vi "WSVCAP SHL Host LL Build SRL Set Voltage CMD.vi"(5 "Data out (14-bit)":u16 format="%04x", 6 "FPGA (Required for Vref = -1)":T1, 7 "Vref (-1: Unchanged)":dbl=-1.0 format="%.3f V", 8 "error in (no error)":errorcluster, 9 "Voltage (-1: Use Data Out)":dbl=-1.0 format="%.3f V", 10 "Channel (0-5)":u32, 11 "DUT":T2) -> (0 "error out":errorcluster, 1 "Raw CMD [Hex]":u32 max=5 step=1 format="0x%05x", 2 "Dev Idx (0-5)":u32, 3 "Raw CMD [Str]":string, 4 "Device Ch Idx (0-31)":u32)   [LabVIEW 2017]
uses:
  Type Defs/WSVCAP SHL DUT Number Enum.ctl
  Type Defs/WSVCAP SHL FPGA Enum.ctl
  Host SRL/Host SRL.lvlib
panel:
  out "Vref Used (V)":dbl format="%.3f V"
  out "D [U16]":u32 format="%.0x"
  out "Raw CMD [Bin]":u32 max=5 step=1 format="0b%019b"
  # "D = [Vout * (2^14)] / (50 * Vref)"
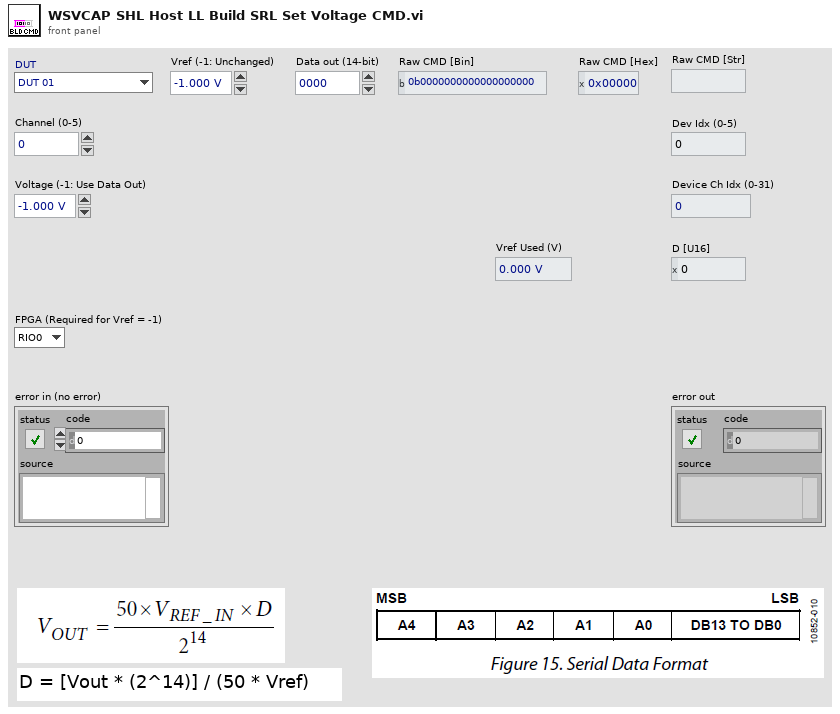
[diagram p1: front panel]
types:
  T1 = typedef "WSVCAP SHL FPGA Enum.ctl" = enum16{"RIO0", "RIO1"}
  T2 = typedef "WSVCAP SHL DUT Number Enum.ctl" = enum16{"DUT 01", "DUT 02", "DUT 03", "DUT 04", "DUT 05", "DUT 06", "DUT 07", "DUT 08", "DUT 09", "DUT 10", "DUT 11", "DUT 12", "DUT 13", "DUT 14", "DUT 15", "DUT 16", "DUT 17", "DUT 18", "DUT 19", "DUT 20", "DUT 21", "DUT 22", "DUT 23", "DUT 24"}
  T3 = typedef "WSVCAP SHL Core System Cluster.ctl" = cluster{"Settings":T4, "FPGA Resource":tag, "Online":bool, "I2C Wait Ticks":u32, "SRL Wait Ticks":u32, "FPGA VI Reference (FPGA Mode)":T5, "FPGA VI Reference (Sim Mode)":refnum<vi>}
  T4 = typedef "WSVCAP SHL I2C Settings Cluster.ctl" = cluster{"I2C Slave Address":u8, "I2C Clock Rate (Hz)":dbl, "SRL Clock Rate (Hz)":dbl, "Simulate FPGA":bool, "C1 Cap DAC Default":u8, "C2 Cap DAC Default":u8, "C3 Cap DAC Default":u8, "C4 Cap DAC Default":u8, "DAC Out Vref (V)":dbl}
  T5 = typedef "WSVCAP SHL FPGA Ref.ctl" = refnum<k20>
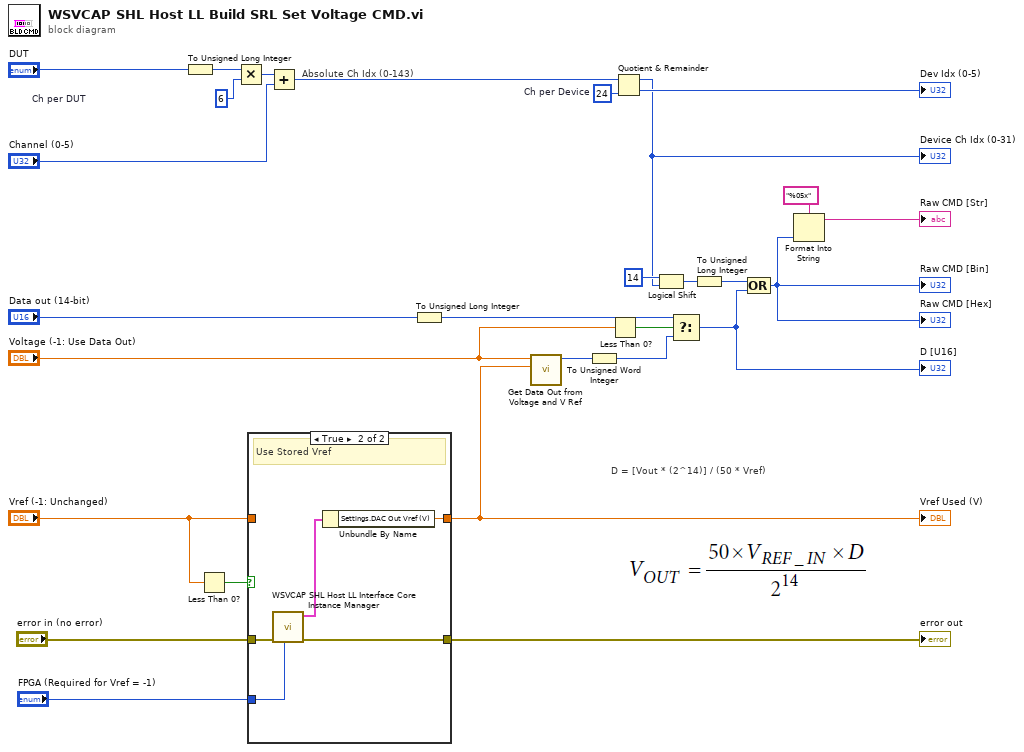
[diagram p0: block diagram]
diagram:
  w18 = u32 6  # Ch per DUT
  w21 = u32 24  # Ch per Device
  # "Absolute Ch Idx (0-143)"
  # "D = [Vout * (2^14)] / (50 * Vref)"
  n1 = To Unsigned Long Integer(number="DUT") -> (unsigned 32bit integer=w19:u32)
  n2 = Less Than 0?(x="Vref (-1: Unchanged)") -> (x < 0?=w9:bool)
  n3 = Multiply(x=w19, y=w18) -> (x*y=w17:u32)
  n4 = case shown="True" w9 {
    tunnel: "FPGA (Required for Vref = -1)" -> [_ w35]
    tunnel: "error in (no error)" -> [w29 w33]
    tunnel: [w29 w32] -> w11
    tunnel: [w30 w31] -> w10
    tunnel: "Vref (-1: Unchanged)" -> [w30 _]
    frame False {
      # "Use Vref Input"
    }
    frame True {
      # "Use Stored Vref"
      n5 = call "WSVCAP SHL Host LL Interface Core Instance Manager.vi"("FPGA"=w35, "error in (no error)"=w33) -> ("error out"=w32:errorcluster, "FGPA Interface Out"=w34:T3)  [unwired: 8 in]
      n6 = Unbundle By Name(w34) -> ("Settings.DAC Out Vref (V)"=w31:dbl)
    }
  }
  "Vref Used (V)" <- w10
  "error out" <- w11
  n7 = Add(x=w17, y="Channel (0-5)") -> (x+y=w15:u32)
  n8 = To Unsigned Long Integer(number="Data out (14-bit)") -> (unsigned 32bit integer=w4:u32)
  n9 = call "Get Data Out from Voltage and V Ref.vi"("Vref (V)"=w10, "Voltage (V)"="Voltage (-1: Use Data Out)") -> ("Data Out (14-bit)"=w3:u16)  [unwired: 9 in]
  n10 = To Unsigned Word Integer(number=w3) -> (unsigned 16bit integer=w1:u16)
  n11 = Less Than 0?(x="Voltage (-1: Use Data Out)") -> (x < 0?=w6:bool)
  n12 = Quotient & Remainder(x=w15, y=w21) -> (x-y*floor(x/y)=w14:u32, floor(x/y)=→"Dev Idx (0-5)":u32)
  "Device Ch Idx (0-31)" <- w14
  n13 = Logical Shift(y=i16 14, x=w14) -> (x << y=w27:u32)
  n14 = Select(t=w4, s=w6, f=w1) -> (s? t:f=w2:u32)
  "D [U16]" <- w2
  n15 = To Unsigned Long Integer(number=w27) -> (unsigned 32bit integer=w26:u32)
  n16 = Compound Arithmetic op=OR(w26, w2) -> (w25:u32)
  "Raw CMD [Bin]" <- w25
  "Raw CMD [Hex]" <- w25
  n17 = Format Into String(format string="%05x", w25) -> (resulting string=→"Raw CMD [Str]":string)  [unwired: 2 in, 1 out]
